vi "SSC Digital Configure Time Set Drive Format.vi"(0 "Digital SSC in":T2[](array[typedef]), 5 "time set":string caption="Time Set", 7 "format":T1=1500 items=["Non-Return"=1500, "Return-to-Low"=1501, "Return-to-High"=1502, "Surround-by-Complement"=1503], 11 "error in":errorcluster) -> (4 "Digital SSC out":T2[](array[typedef]), 15 "error out":errorcluster)   [LabVIEW 2019]
doc: "Configures the tset edge. \nBelow are the corresponding property from mflex code.\n\n• chEdgeD0: Drive On \n• chEdgeD1: Drive Data \n• chEdgeD2: Drive Return \n• chEdgeD3: Drive Off \n• chEdgeR0: Compare Open \n• chEdgeR1: Compare Close"
uses:
  SSC Digital.ctl
  <instrlib>/niDigital/niDigital.llb/niDigital Drive Format.ctl
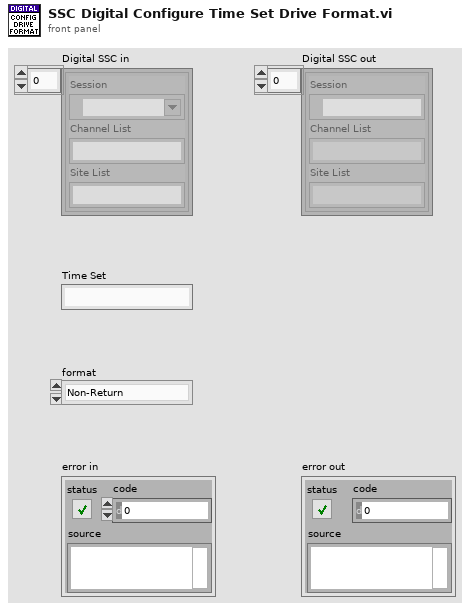
[diagram p1: front panel]
types:
  T1 = typedef "niDigital Drive Format.ctl" = i32
  T2 = typedef "SSC Digital.ctl" = cluster{"Session":refnum<k15>, "Channel List":string, "Site List":string}
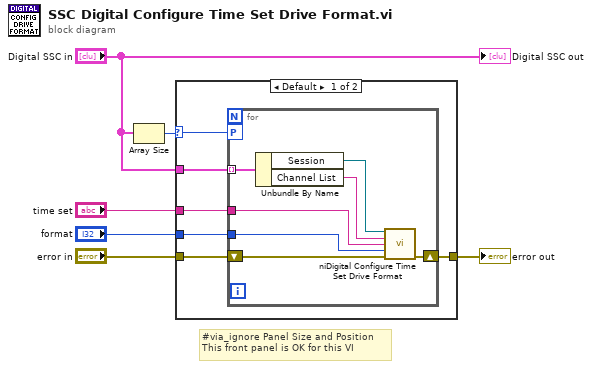
[diagram p0: block diagram]
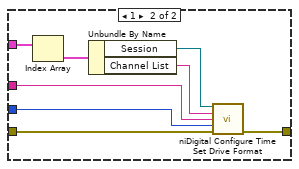
[diagram p2: hidden frame]
diagram:
  # "#via_ignore Panel Size and Position\nThis front panel is OK for this VI"
  n1 = Array Size(array="Digital SSC in") -> (size(s)=w4:i32)
  n2 = case shown="Default" w4 {
    selector: w4 -> [w12 _]
    tunnel: "error in" -> [w10 w24]
    tunnel: [w8 w25] -> w5
    tunnel: "Digital SSC in" -> [w11 w27]
    tunnel: "time set" -> [w9 w21]
    tunnel: "format" -> [w7 w20]
    frame Default {
      n3 = for {
        workers-P: w12 -> [_]
        tunnel: w11 -> [w19] mode=indexing
        tunnel: w9 -> [w14]
        shift-right: [w17] -> w8
        shift-left: w10 -> [w18]
        tunnel: w7 -> [w13]
        n4 = Unbundle By Name(w19) -> ("Session"=w16:refnum<k15>, "Channel List"=w15:string)
        n5 = call <instrlib>:"niDigital Configure Time Set Drive Format.vi"("instrument handle"=w16, "pin list"=w15, "time set"=w14, "format"=w13, "error in"=w18) -> ("error out"=w17:errorcluster)  [unwired: 9 in, 1 out]
      }
    }
    frame 1 {
      n6 = Index Array(array=w27) -> (element=w26:T2)  [unwired: 1 in]
      n7 = Unbundle By Name(w26) -> ("Session"=w23:refnum<k15>, "Channel List"=w22:string)
      n8 = call <instrlib>:"niDigital Configure Time Set Drive Format.vi"("instrument handle"=w23, "pin list"=w22, "time set"=w21, "format"=w20, "error in"=w24) -> ("error out"=w25:errorcluster)  [unwired: 9 in, 1 out]
    }
  }
  "error out" <- w5
  "Digital SSC out" <- "Digital SSC in"
